vi "Test MB7047 I2C Sensors.vi"() -> ()   [LabVIEW 2011]
uses:
  <vilib>/LabVIEW Interface for Arduino/LabVIEW Interface for Arduino.lvlib
panel:
  in  "Wait for Reading":u32=100
  out "concatenated string":string
  out "I2C Data 3":u8[](array[numeric]) format="%x"
  out "Slide 3":u8(slide) scale=0.0..300.0
  out "floor(x/y) 3":u32
  in  "Delay (ms)":u32=100
  out "floor(x/y)":u32
  out "Slide":u8(slide) scale=0.0..300.0
  out "I2C Data":u8[](array[numeric]) format="%x"
  out "I2C Data 2":u8[](array[numeric]) format="%x"
  out "Slide 2":u8(slide) scale=0.0..300.0
  out "floor(x/y) 2":u32
  in  "stop":bool
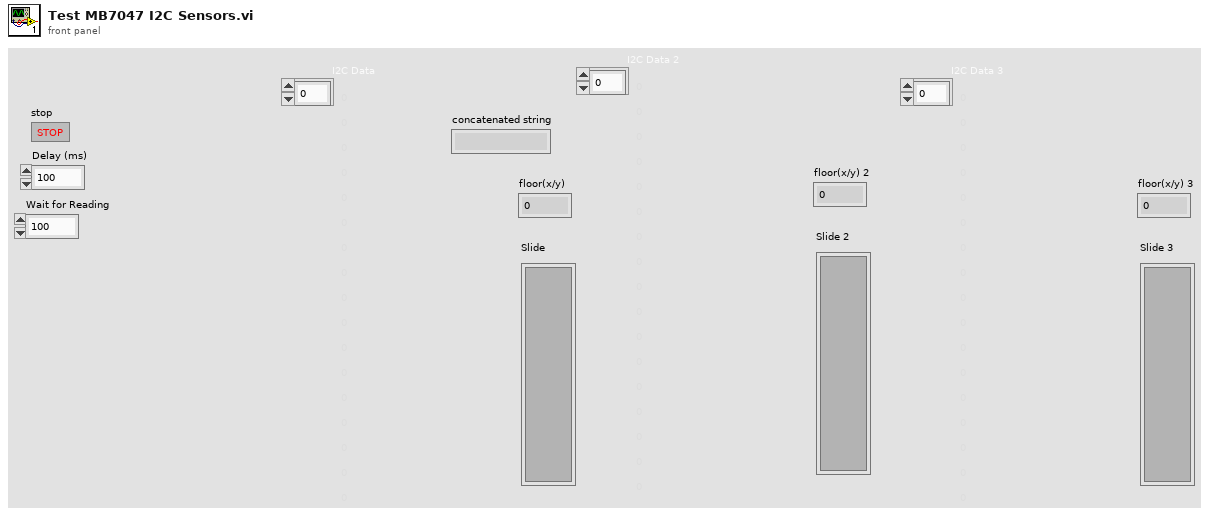
[diagram p1: front panel]
types:
  T1 = typedef "LabVIEW Interface for Arduino.lvlib/Arduino Resource.ctl" = cluster{"VISA resource":refnum<visa-resource-name>, "Board Type":T2, "Connection Type":enum8{"USB / Serial"}, "Bytes Per Packet (15)":u8}
  T2 = typedef "LabVIEW Interface for Arduino.lvlib/Board Type.ctl" = enum16{"Uno", "Dimuelanove w/Atmega 328", "Mega 2560"}
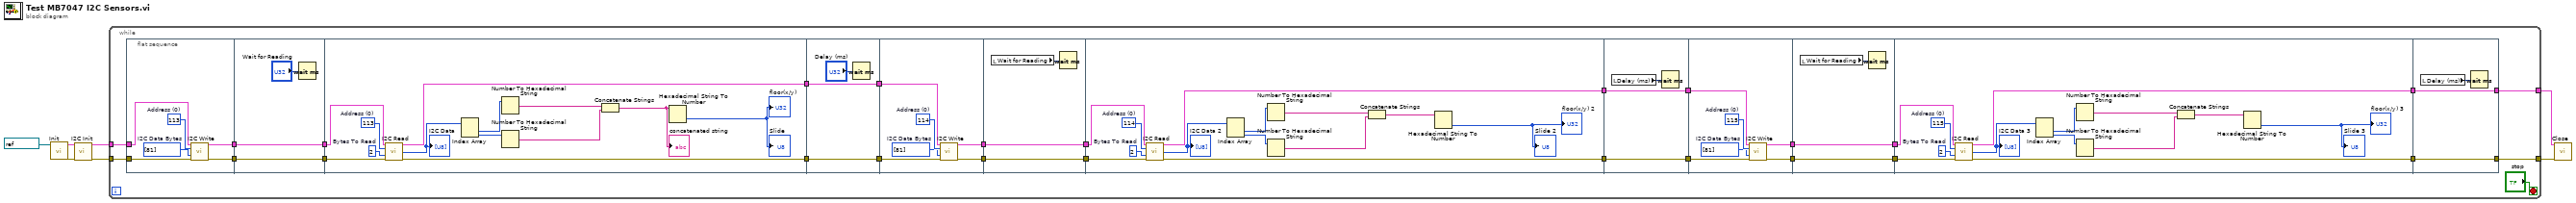
[diagram p0: block diagram]
diagram:
  n1 = call <vilib>:"Init.vi"("VISA resource"=refnum<visa-resource-name> "COM4") -> ("Arduino Resource"=w7:T1, "error out"=w6:errorcluster)  [unwired: 17 in]
  n2 = call <vilib>:"I2C Init.vi"("Arduino Resource"=w7, "error in"=w6) -> ("Arduino Resource"=w5:T1, "error out"=w4:errorcluster)  [unwired: 12 in]
  n3 = while {
    tunnel: w5 -> [w34]
    tunnel: w4 -> [w33]
    tunnel: [w32] -> w3
    tunnel: [w31] -> w2
    stop <- "stop" stop-if-true
    n4 = flat-sequence {
      tunnel: w34 -> [w40]
      tunnel: w33 -> [w39]
      tunnel: [w37] -> w30
      tunnel: [w36] -> w29
      tunnel: [w43] -> w25
      tunnel: w30 -> [w43]
      tunnel: [w42] -> w24
      tunnel: w29 -> [w42]
      tunnel: w25 -> [w47]
      tunnel: [w45] -> w21
      tunnel: w24 -> [w46]
      tunnel: [w44] -> w19
      tunnel: w21 -> [w59]
      tunnel: [w59] -> w20
      tunnel: w19 -> [w58]
      tunnel: [w58] -> w18
      tunnel: w20 -> [w63]
      tunnel: [w61] -> w27
      tunnel: w18 -> [w62]
      tunnel: [w60] -> w26
      tunnel: w27 -> [w68]
      tunnel: w26 -> [w67]
      tunnel: [w68] -> w23
      tunnel: [w67] -> w22
      tunnel: w23 -> [w72]
      tunnel: w22 -> [w71]
      tunnel: [w70] -> w13
      tunnel: [w69] -> w11
      tunnel: w13 -> [w84]
      tunnel: [w84] -> w12
      tunnel: w11 -> [w83]
      tunnel: [w83] -> w10
      tunnel: [w87] -> w15
      tunnel: w12 -> [w88]
      tunnel: w10 -> [w86]
      tunnel: [w85] -> w8
      tunnel: w15 -> [w93]
      tunnel: [w93] -> w14
      tunnel: [w92] -> w9
      tunnel: w8 -> [w92]
      tunnel: [w96] -> w17
      tunnel: w14 -> [w95]
      tunnel: [w97] -> w16
      tunnel: w9 -> [w94]
      tunnel: [w108] -> w31
      tunnel: [w109] -> w32
      tunnel: w17 -> [w109]
      tunnel: w16 -> [w108]
      frame #0 {
        w38 = u8[] [81]  # I2C Data Bytes
        w35 = u8 113  # Address (0)
        n5 = call <vilib>:"I2C Write.vi"("Arduino Resource"=w40, "Address (0)"=w35, "I2C Data Bytes"=w38, "error in"=w39) -> ("Arduino Resource"=w37:T1, "error out"=w36:errorcluster)  [unwired: 10 in]
      }
      frame #1 {
        n6 = Wait (ms)(milliseconds to wait="Wait for Reading") -> ()  [unwired: 1 out]
      }
      frame #2 {
        w48 = u8 113  # Address (0)
        w56 = u8 2  # Bytes To Read
        n7 = call <vilib>:"I2C Read.vi"("Arduino Resource"=w47, "Address (0)"=w48, "Bytes To Read"=w56, "error in"=w46) -> ("Arduino Resource"=w45:T1, "I2C Data"=w50:u8[], "error out"=w44:errorcluster)  [unwired: 9 in]
        "I2C Data" <- w50
        n8 = Index Array "Index Array"(array=w50) -> (element #1=w51:u8, element #2=w52:u8)  [unwired: 2 in]
        n9 = Number To Hexadecimal String(2:w51) -> (0:w54:string)  [unwired: 1 out]
        n10 = Number To Hexadecimal String(2:w52) -> (0:w53:string)  [unwired: 1 out]
        n11 = Concatenate Strings "Concatenate Strings"(w54, w53) -> (w55:string)
        "concatenated string" <- w55
        n12 = Hexadecimal String To Number(string=w55) -> (number=→"Slide" →"floor(x/y)":u32)  [unwired: 3 out]
      }
      frame #3 {
        n13 = Wait (ms)(milliseconds to wait="Delay (ms)") -> ()  [unwired: 1 out]
      }
      frame #4 {
        w64 = u8[] [81]  # I2C Data Bytes
        w65 = u8 114  # Address (0)
        n14 = call <vilib>:"I2C Write.vi"("Arduino Resource"=w63, "Address (0)"=w65, "I2C Data Bytes"=w64, "error in"=w62) -> ("Arduino Resource"=w61:T1, "error out"=w60:errorcluster)  [unwired: 10 in]
      }
      frame #5 {
        n15 = local read "Wait for Reading"() -> (w66:u32)
        n16 = Wait (ms)(milliseconds to wait=w66) -> ()  [unwired: 1 out]
      }
      frame #6 {
        w81 = u8 114  # Address (0)
        w73 = u8 2  # Bytes To Read
        n17 = call <vilib>:"I2C Read.vi"("Arduino Resource"=w72, "Address (0)"=w81, "Bytes To Read"=w73, "error in"=w71) -> ("Arduino Resource"=w70:T1, "I2C Data"=w79:u8[], "error out"=w69:errorcluster)  [unwired: 9 in]
        "I2C Data 2" <- w79
        n18 = Index Array "Index Array"(array=w79) -> (element #1=w78:u8, element #2=w77:u8)  [unwired: 2 in]
        n19 = Number To Hexadecimal String(2:w78) -> (0:w75:string)  [unwired: 1 out]
        n20 = Number To Hexadecimal String(2:w77) -> (0:w76:string)  [unwired: 1 out]
        n21 = Concatenate Strings "Concatenate Strings"(w75, w76) -> (w74:string)
        n22 = Hexadecimal String To Number(string=w74) -> (number=→"Slide 2" →"floor(x/y) 2":u32)  [unwired: 3 out]
      }
      frame #7 {
        n23 = local read "Delay (ms)"() -> (w82:u32)
        n24 = Wait (ms)(milliseconds to wait=w82) -> ()  [unwired: 1 out]
      }
      frame #8 {
        w89 = u8[] [81]  # I2C Data Bytes
        w90 = u8 115  # Address (0)
        n25 = call <vilib>:"I2C Write.vi"("Arduino Resource"=w88, "Address (0)"=w90, "I2C Data Bytes"=w89, "error in"=w86) -> ("Arduino Resource"=w85:T1, "error out"=w87:errorcluster)  [unwired: 10 in]
      }
      frame #9 {
        n26 = local read "Wait for Reading"() -> (w91:u32)
        n27 = Wait (ms)(milliseconds to wait=w91) -> ()  [unwired: 1 out]
      }
      frame #10 {
        w98 = u8 115  # Address (0)
        w106 = u8 2  # Bytes To Read
        n28 = call <vilib>:"I2C Read.vi"("Arduino Resource"=w94, "Address (0)"=w98, "Bytes To Read"=w106, "error in"=w95) -> ("Arduino Resource"=w96:T1, "I2C Data"=w100:u8[], "error out"=w97:errorcluster)  [unwired: 9 in]
        "I2C Data 3" <- w100
        n29 = Index Array "Index Array"(array=w100) -> (element #1=w101:u8, element #2=w102:u8)  [unwired: 2 in]
        n30 = Number To Hexadecimal String(2:w101) -> (0:w104:string)  [unwired: 1 out]
        n31 = Number To Hexadecimal String(2:w102) -> (0:w103:string)  [unwired: 1 out]
        n32 = Concatenate Strings "Concatenate Strings"(w104, w103) -> (w105:string)
        n33 = Hexadecimal String To Number(string=w105) -> (number=→"Slide 3" →"floor(x/y) 3":u32)  [unwired: 3 out]
      }
      frame #11 {
        n34 = local read "Delay (ms)"() -> (w107:u32)
        n35 = Wait (ms)(milliseconds to wait=w107) -> ()  [unwired: 1 out]
      }
    }
  }
  n36 = call <vilib>:"Close.vi"("Arduino Resource"=w3, "error in"=w2) -> ()  [unwired: 13 in, 1 out]
